vi "Read Absolute Pressure.vi"(8 "error in (no error)":errorcluster, 11 "VISA resource name":refnum<visa-resource-name>) -> (0 "error out":errorcluster, 1 "Downstream Absolute Pressure":dbl, 2 "Upstream Absolute Pressure":dbl, 3 "VISA resource name out":refnum<visa-resource-name>)   [LabVIEW 2023, in "Fluke Molbox 1 Plus.lvlib"]
doc: "Reads the last measured absolute pressure both downstream and upstream.\n\n<B>Note:</B>\nThe current pressure value is returned in the current pressure unit of measure."
uses:
  Fluke Molbox 1 Plus.lvlib
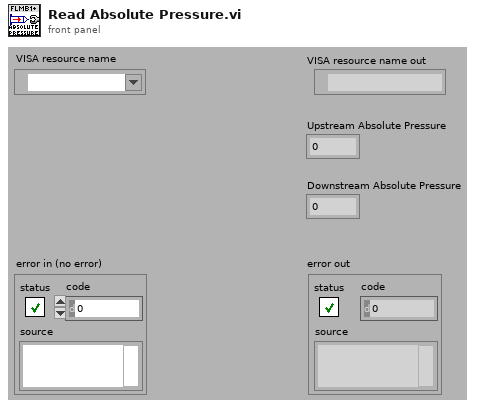
[diagram p1: front panel]
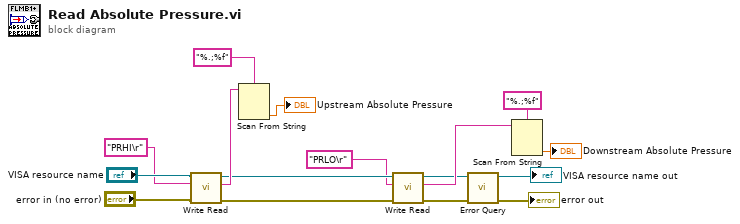
[diagram p0: block diagram]
diagram:
  n1 = call "Write Read.vi"("error in (no error)"="error in (no error)", "Write String"="PRHI\r" ("write buffer"), "VISA resource name"="VISA resource name") -> ("error out"=w7:errorcluster, "Read Response"=w9:string, "VISA resource name out"=w8:refnum<visa-resource-name>)  [unwired: 6 in]
  n2 = Scan From String(format string="%.;%f", input string=w9) -> (output 1=→"Upstream Absolute Pressure":dbl)  [unwired: 3 in, 3 out]
  n3 = call "Write Read.vi"("error in (no error)"=w7, "Write String"="PRLO\r" ("write buffer"), "VISA resource name"=w8) -> ("error out"=w3:errorcluster, "Read Response"=w6:string, "VISA resource name out"=w4:refnum<visa-resource-name>)  [unwired: 6 in]
  n4 = call "Error Query.vi"("error in (no error)"=w3, "VISA resource name"=w4) -> ("error out"=→"error out":errorcluster, "VISA resource name out"=→"VISA resource name out":refnum<visa-resource-name>)  [unwired: 6 in, 2 out]
  n5 = Scan From String(format string="%.;%f", input string=w6) -> (output 1=→"Downstream Absolute Pressure":dbl)  [unwired: 3 in, 3 out]
